vi "Set Attribute STRING.vi"(8 "error in":errorcluster, 9 "Value":string, 10 "Path":string, 11 "Config from JSON in":refnum<class "Config from JSON.lvclass">) -> (0 "error out":errorcluster, 3 "Config from JSON out":refnum<class "Config from JSON.lvclass">)   [LabVIEW 2025, in "Config from JSON.lvclass"]
uses:
  Config from JSON.lvclass
  Config from JSON.lvclass/Config from JSON.ctl
  791a158e-6076-414b-849b-f128768fad82.vi
  <vilib>/JDP Science/JSONtext/Variant to JSON Text.vi
  <vilib>/JDP Science/JSONtext/Set Item.vi
  <vilib>/JDP Science/JSONtext/LVClass Serializer/JSONtext LVClass Serializer.lvclass
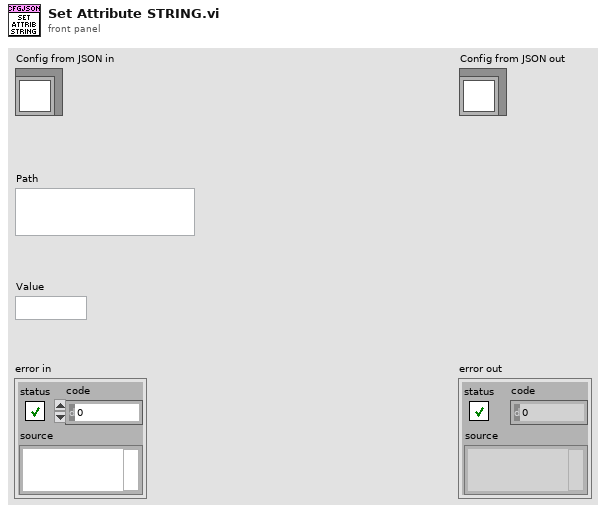
[diagram p1: front panel]
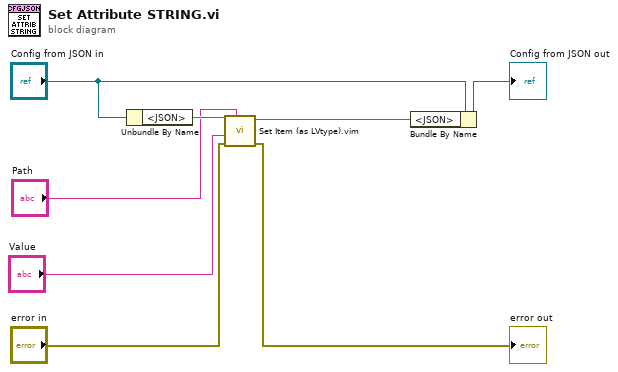
[diagram p0: block diagram]
diagram:
  n1 = Unbundle By Name("Config from JSON in") -> ("<JSON>"=w7:string)
  n2 = call "Set Item (as LVtype).vim"("$Path or Item Name"="Path", "error in (no error)"="error in", "Anything"="Value", "JSON"=w7) -> ("error out"=→"error out":errorcluster, "<JSON>"=w5:string)  [unwired: 4 in, 1 out]
  n3 = Bundle By Name(cluster="Config from JSON in", "<JSON>"=w5) -> (→"Config from JSON out":refnum<class "Config from JSON.lvclass">)
